vi "ReplaceDots.vi"(8 "error in":errorcluster, 10 "search string":string=".", 11 "String In":string) -> (0 "error out":errorcluster, 3 "String Out":string)   [LabVIEW 2022 SP3]
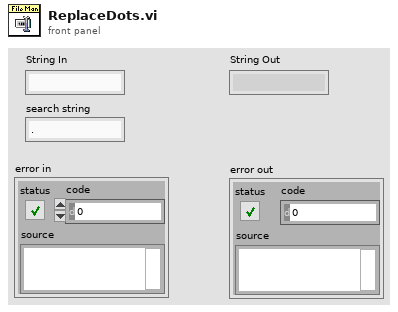
[diagram p1: front panel]
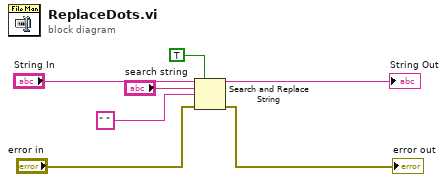
[diagram p0: block diagram]
diagram:
  n1 = Search and Replace String(replace all?=TRUE ("replace all? (F)"), input string="String In", search string="search string", replace string=" " ("replace string (\"\")"), error in="error in") -> (result string=→"String Out":string, error out=→"error out":errorcluster)  [unwired: 3 in, 2 out]
